vi "Calc Currente Exposure Time.vi"(8 "error in (no error)":errorcluster, 11 "CCDCamera in":refnum<class "CCDCamera.lvclass">) -> (0 "error out":errorcluster, 3 "CCDCamera out":refnum<class "CCDCamera.lvclass">)   [LabVIEW 2018, in "CCDCamera.lvclass"]
uses:
  CCDCamera.lvclass
  CCDCamera.lvclass/CCDCamera.ctl
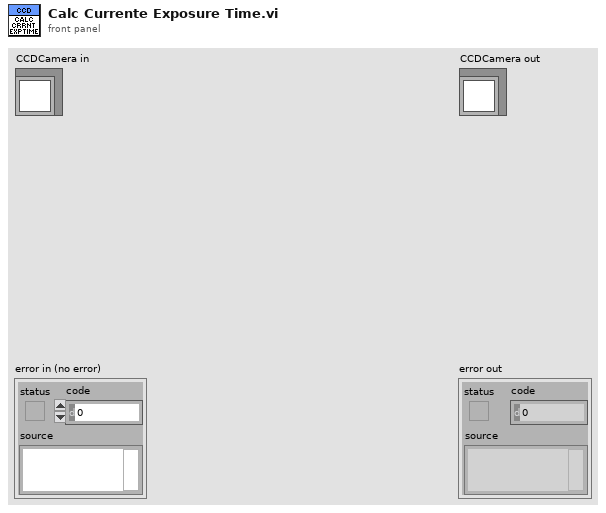
[diagram p1: front panel]
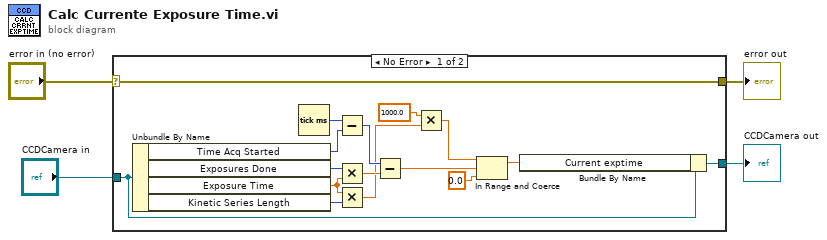
[diagram p0: block diagram]
diagram:
  n1 = case shown="No Error" "error in (no error)" {
    selector: "error in (no error)" -> [w20 w22]
    tunnel: [w20 w22] -> w3
    tunnel: [w16 w21] -> w1
    tunnel: "CCDCamera in" -> [w17 w21]
    frame No Error {
      n2 = Unbundle By Name(w17) -> ("Time Acq Started"=w18:u32, "Exposures Done"=w15:u16, "Exposure Time"=w12:sgl, "Kinetic Series Length"=w11:u32)
      n3 = Tick Count (ms)() -> (millisecond timer value=w19:u32)
      n4 = Subtract(x=w19, y=w18) -> (x-y=w14:u32)
      n5 = Multiply(x=w15, y=w12) -> (x*y=w13:sgl)
      n6 = Multiply(x=w12, y=w11) -> (x*y=w7:sgl)
      n7 = Subtract(x=w14, y=w13) -> (x-y=w9:sgl)
      n8 = Multiply(x=sgl 1000.0, y=w7) -> (x*y=w6:sgl)
      n9 = In Range and Coerce(upper limit=w6, x=w9, lower limit=sgl 0.0) -> (coerced(x)=w8:sgl)  [unwired: 1 out]
      n10 = Bundle By Name(cluster=w17, "Current exptime"=w8) -> (w16:refnum<class "CCDCamera.lvclass">)
    }
    frame Error {
    }
  }
  "error out" <- w3
  "CCDCamera out" <- w1
